vi "Block Name to Paths.vi"(10 "Block Name":string) -> (2 "Image Path":path, 3 "Block Path":path)   [LabVIEW 2024]
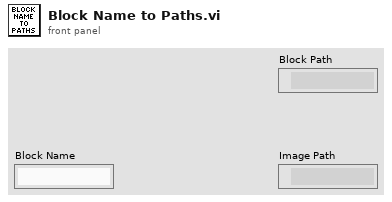
[diagram p1: front panel]
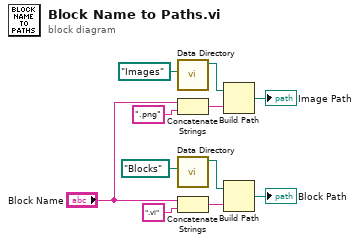
[diagram p0: block diagram]
diagram:
  n1 = call "Data Directory.vi"("Subdirectory"=path "Images" ("name or relative path")) -> ("Data directory"=w2:path)  [unwired: 9 in, 1 out]
  n2 = Concatenate Strings("Block Name", ".png" ("string")) -> (w7:string)
  n3 = call "Data Directory.vi"("Subdirectory"=path "Blocks" ("name or relative path")) -> ("Data directory"=w3:path)  [unwired: 9 in, 1 out]
  n4 = Concatenate Strings("Block Name", ".vi" ("string")) -> (w11:string)
  n5 = Build Path(base path=w2, name or relative path=w7) -> (appended path=→"Image Path":path)
  n6 = Build Path(base path=w3, name or relative path=w11) -> (appended path=→"Block Path":path)
